vi "In Range & Coerce.vi"() -> ()   [LabVIEW 2016]
panel:
  in  "Numeric 4":dbl
  out "Boolean":bool
  out "Numeric 3":dbl
  in  "Numeric 2":dbl
  in  "Numeric":dbl
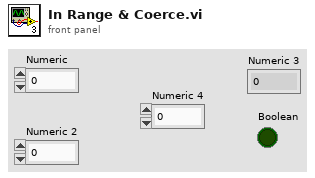
[diagram p1: front panel]
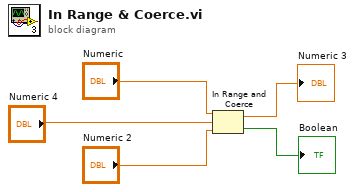
[diagram p0: block diagram]
diagram:
  n1 = In Range and Coerce(upper limit="Numeric", x="Numeric 4", lower limit="Numeric 2") -> (coerced(x)=→"Numeric 3":dbl, In Range?=→"Boolean":bool)
